vi "PH_DataViewer.destructor.vi"(0 "i ref in":refnum<vi>, 5 "error in(no error)":errorcluster) -> (19 "error out":errorcluster)   [LabVIEW 2014, in "PH_DataViewer.lvlib"]
doc: "This is the destructor of a class.\n\nLicense Agreement for this software:\n\nCopyright (C)\nGesellschaft für Schwerionenforschung, GSI\nPlanckstr. 1\n64291 Darmstadt\nGermany\n\nContact: D.Beck@gsi.de \n\nThis program is free software; you can redistribute it and/or modify it under the terms of the \nGNU General Public License as published by the Free Software Foundation; either version 2 of \nthe license, or (at your option) any later version.\n\nThis program is distributed in the hope that it will be useful, but WITHOUT ANY WARRANTY; \nwithout even the implied warranty of MERCHANTABILITY or FITNESS FOR A PARTICULAR PURPOSE. See the GNU General License for more details (http://www.gnu.org).\n\nGesellschaft für Schwerionenforschung, GSI\nPlanckstr. 1, 64291 Darmstadt, Germany\nFor all questions and ideas contact: M.Richter@gsi.de, H.Brand@gsi.de or D.Beck@gsi.de.\nLast update: 16-JUN-2004"
uses:
  PH_DataViewer.lvlib
  CSCore/BaseGUI/BaseGUI.lvlib
  CSCore/CSObj/CSObj.lvlib
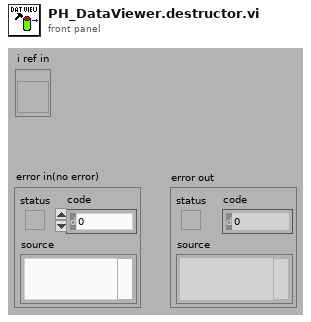
[diagram p1: front panel]
types:
  T1 = enum16{"SetAttribute", "GetAttribute", "CreateAttribute", "DestroyAttribute", "DestroyAllAtributes"}
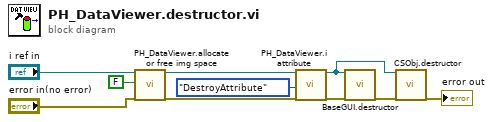
[diagram p0: block diagram]
diagram:
  n1 = call "PH_DataViewer.allocate or free img space.vi"("i ref in"="i ref in", "Allocate?"=FALSE, "error in (no error)"="error in(no error)") -> ("i ref out"=w5:refnum<vi>, "error out"=w7:errorcluster)  [unwired: 15 in]
  n2 = call "PH_DataViewer.i attribute.vi"("VI Refnum"=w5, "Action"=T1."DestroyAttribute", "error in (no error)"=w7) -> ("VI Refnum out"=w1:refnum<vi>, "error out"=w9:errorcluster)  [unwired: 14 in, 1 out]
  n3 = call "BaseGUI.destructor.vi"("i ref in"=w1, "error in (no error)"=w9) -> ("error out"=w3:errorcluster)  [unwired: 17 in]
  n4 = call "CSObj.destructor.vi"("i ref in"=w1, "error in (no error)"=w3) -> ("error out"=→"error out":errorcluster)  [unwired: 17 in]
